vi "Save Fuel State.vi"(8 "error in":errorcluster, 10 "Slave ID":dbl, 11 "Session in":refnum<class "MB_Master.lvclass">) -> (0 "error out":errorcluster)   [LabVIEW 2017, in "Akwizycja.lvlib"]
uses:
  Akwizycja.lvlib
  <vilib>/Plasmionique/MB Master/MB_Master/MB_Master.lvclass
  <vilib>/Utility/config.llb/NI_LVConfig.lvlib
  <vilib>/Plasmionique/MB Master/MB Master.lvlib
panel:
  in  "Px":T1
  in  "?":T2
  in  "?":T2
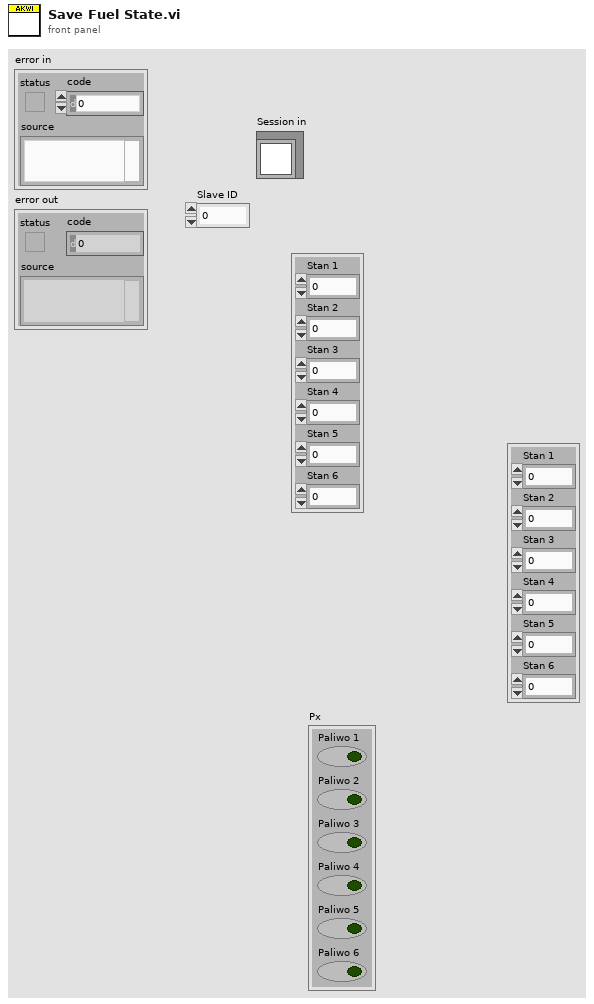
[diagram p1: front panel]
types:
  T1 = cluster{"Paliwo 1":bool, "Paliwo 2":bool, "Paliwo 3":bool, "Paliwo 4":bool, "Paliwo 5":bool, "Paliwo 6":bool}
  T2 = cluster{"Stan 1":dbl, "Stan 2":dbl, "Stan 3":dbl, "Stan 4":dbl, "Stan 5":dbl, "Stan 6":dbl}
  T3 = typedef "NI_LVConfig.lvlib/Config Data RefNum.ctl" = refnum<k1>
  T4 = cluster{"[0]":dbl, "[1]":dbl, "[2]":dbl, "[3]":dbl, "[4]":dbl, "[5]":dbl}
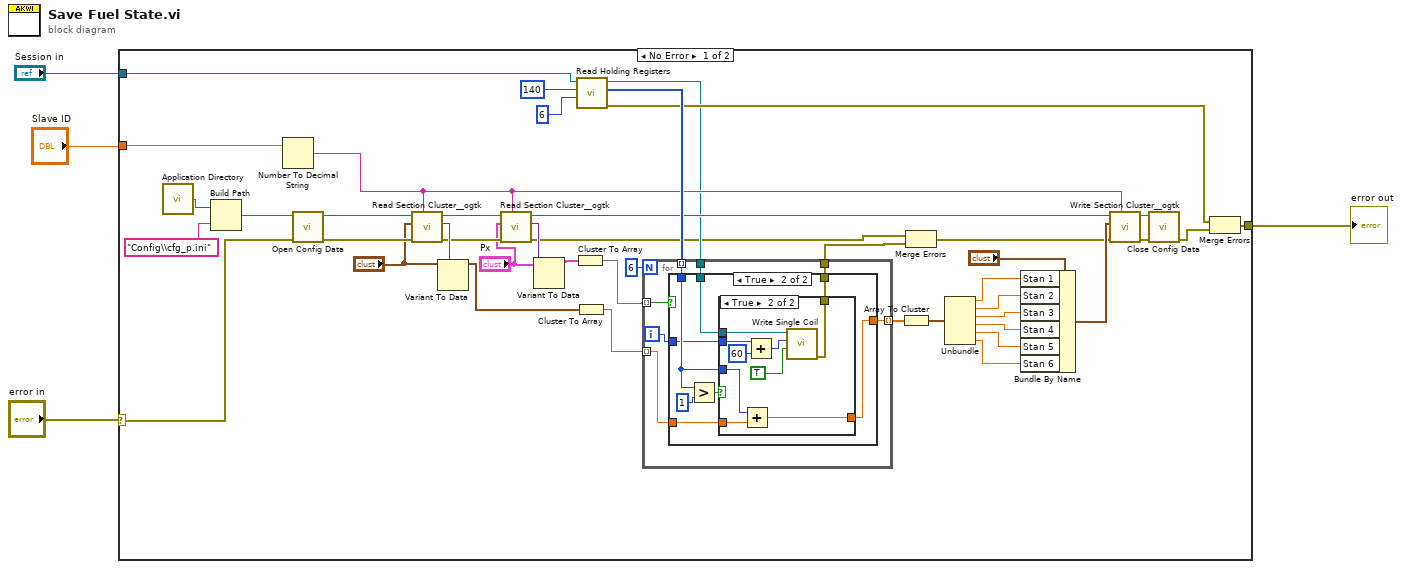
[diagram p0: block diagram]
diagram:
  n1 = case shown="No Error" "error in" {
    selector: "error in" -> [w18 w74]
    tunnel: "Slave ID" -> [w39 _]
    tunnel: [w19 w74] -> w3
    tunnel: "Session in" -> [w17 _]
    frame No Error {
      n2 = call <vilib>:"Application Directory.vi"() -> ("Application Directory"=w47:path)
      n3 = Build Path(base path=w47, name or relative path="Config\\cfg_p.ini") -> (appended path=w45:path)
      n4 = Number To Decimal String(number=w39) -> (decimal integer string=w9:string)  [unwired: 1 in]
      n5 = call <vilib>:"Open Config Data.vi"("error in (no error)"=w18, "configuration file path"=w45) -> ("error out"=w43:errorcluster, "refnum"=w42:T3)  [unwired: 7 in, 1 out]
      n6 = call <userlib>:"Read Section Cluster__ogtk.vi"("section (optional)"=w9, "error in (no error)"=w43, "Section Formatted Cluster Type"="?", "refnum"=w42) -> ("error out"=w14:errorcluster, "Section Formatted Cluster"=w36:variant, "dup refnum"=w13:T3)  [unwired: 3 in, 2 out]
      n7 = Variant To Data(type="?", Variant=w36) -> (data=w34:T2)  [unwired: 1 in, 1 out]
      n8 = call <userlib>:"Read Section Cluster__ogtk.vi"("section (optional)"=w9, "error in (no error)"=w14, "Section Formatted Cluster Type"="Px", "refnum"=w13) -> ("error out"=w7:errorcluster, "Section Formatted Cluster"=w12:variant, "dup refnum"=w15:T3)  [unwired: 3 in, 2 out]
      n9 = Variant To Data(type="Px", Variant=w12) -> (data=w11:T1)  [unwired: 1 in, 1 out]
      n10 = Cluster To Array(cluster=w11) -> (array=w35:bool[])
      n11 = Cluster To Array(cluster=w34) -> (array=w33:dbl[])
      n12 = call <vilib>:"Read Holding Registers.vi"("quantity"=u16 6, "starting address"=u16 140, "MB session in"=w17) -> ("error out"=w20:errorcluster, "Registers"=w32:u16[], "MB session out"=w8:refnum<class "MB_Master.lvclass">)  [unwired: 6 in]
      n13 = for {
        N: 6 -> [_]
        tunnel: w35 -> [w54] mode=indexing
        tunnel: w33 -> [w53] mode=indexing
        tunnel: w32 -> [w52] mode=indexing
        tunnel: [w51] -> w31 mode=indexing
        tunnel: w8 -> [w50]
        tunnel: [w48] -> w5
        i -> [w49]
        n14 = case shown="True" w54 {
          tunnel: [w55 w61] -> w51
          tunnel: w53 -> [w55 w62]
          tunnel: w52 -> [_ w60]
          tunnel: w50 -> [_ w58]
          tunnel: w49 -> [_ w57]
          tunnel: [_ w56] -> w48
          frame False {
          }
          frame True {
            n15 = Greater?(x=w60, y=u16 1) -> (0:w59:bool)
            n16 = case shown="True" w59 {
              tunnel: w62 -> [w64 w73]
              tunnel: [w64 w72] -> w61
              tunnel: w60 -> [_ w71]
              tunnel: w58 -> [_ w70]
              tunnel: w57 -> [_ w69]
              tunnel: [_ w65] -> w56
              frame False {
              }
              frame True {
                n17 = Add(x=w71, y=w73) -> (x+y=w72:dbl)
                n18 = Add(x=w69, y=60) -> (x+y=w68:i32)
                n19 = call <vilib>:"Write Single Coil.vi"("value"=TRUE, "address"=w68, "MB session in"=w70) -> ("error out"=w65:errorcluster)  [unwired: 7 in, 1 out]
              }
            }
          }
        }
      }
      n20 = Array To Cluster(array=w31) -> (cluster=w30:T4)
      n21 = Merge Errors(w7, w5) -> (w6:errorcluster)
      n22 = Unbundle(w30) -> ("[0]"=w28:dbl, "[1]"=w27:dbl, "[2]"=w26:dbl, "[3]"=w23:dbl, "[4]"=w24:dbl, "[5]"=w25:dbl)
      n23 = Bundle By Name(cluster="?", "Stan 1"=w28, "Stan 2"=w27, "Stan 3"=w26, "Stan 4"=w23, "Stan 5"=w24, "Stan 6"=w25) -> (w40:T2)
      n24 = call <userlib>:"Write Section Cluster__ogtk.vi"("section (optional)"=w9, "error in (no error)"=w6, "Section Formatted Cluster"=w40, "refnum"=w15) -> ("error out"=w21:errorcluster, "dup refnum"=w44:T3)  [unwired: 6 in]
      n25 = call <vilib>:"Close Config Data.vi"("error in (no error)"=w21, "refnum"=w44) -> ("error out"=w22:errorcluster)  [unwired: 8 in, 1 out]
      n26 = Merge Errors(w20, w22) -> (w19:errorcluster)
    }
    frame Error {
    }
  }
  "error out" <- w3
